vi "DAQ.Init.Override.vi"(8 "error in (no error)":errorcluster, 11 "DAQmx in":refnum<class "DAQmx.lvclass">) -> (0 "error out":errorcluster, 3 "DAQmx out":refnum<class "DAQmx.lvclass">)   [LabVIEW 2016, in "DAQmx.lvclass"]
uses:
  DAQmx.lvclass
  C:/user/patrick/hg/lockin.SMO/lvsrc/DAQ/DAQ.lvclass
  DAQ/DAQ.lvclass/DAQ.ctl
  DAQmx.lvclass/DAQmx.ctl
  <vilib>/DAQmx/write.llb/DAQmx Write (Analog 1D Wfm NChan NSamp).vi
  <vilib>/DAQmx/create/channels.llb/DAQmx Create Channel (AO-Voltage-Basic).vi
  <vilib>/DAQmx/create/channels.llb/DAQmx Create Channel (AI-Voltage-Basic).vi
  <vilib>/DAQmx/configure/timing.llb/DAQmx Timing (Sample Clock).vi
  <vilib>/DAQmx/miscellaneous.llb/DAQmx Fill In Error Info.vi
  <resource>/objmgr/daqmx.rc
  <vilib>/measure/NI_MABase.lvlib
  DAQ/DAQ.lvclass
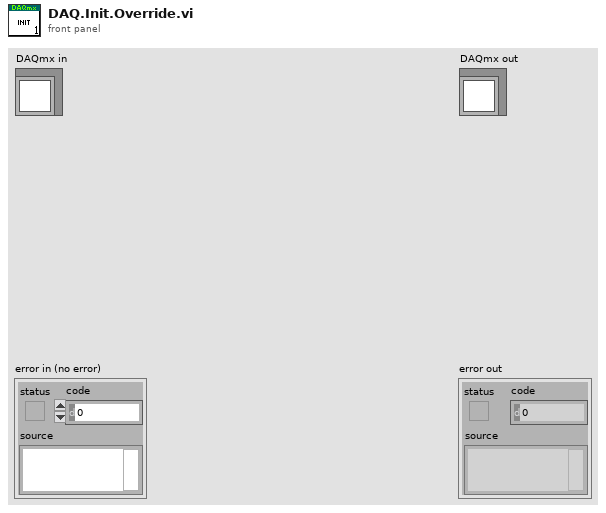
[diagram p1: front panel]
types:
  T1 = typedef "DAQ.lvclass/PrivateEvents--DAQ.AO.Channels.ctl" = string
  T2 = typedef "DAQ.lvclass/PrivateEvents--DAQ.AI.Channels.ctl" = string
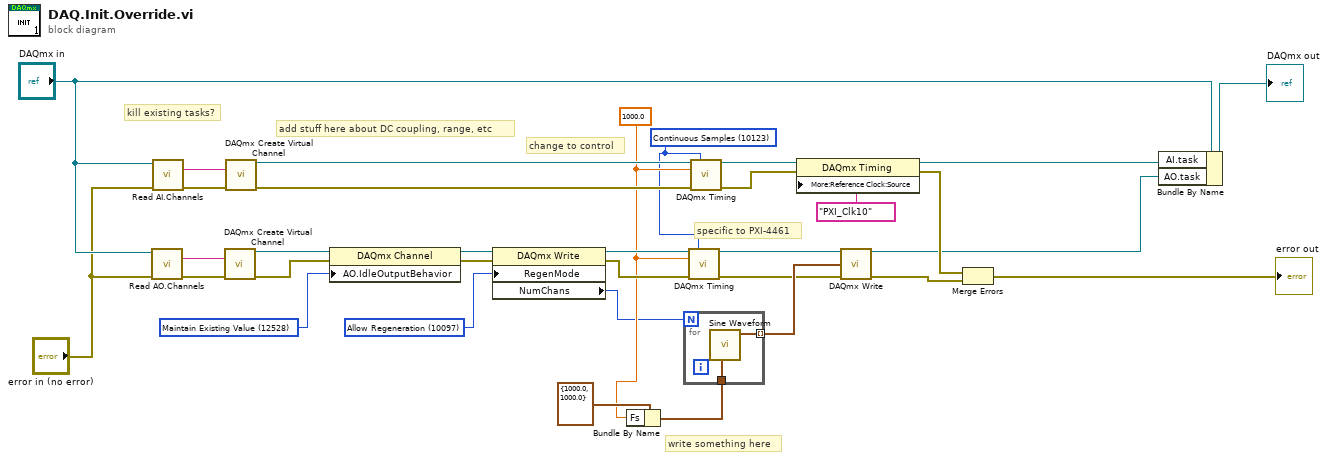
[diagram p0: block diagram]
diagram:
  w1 = 10123 items=["Finite Samples"=10178, "Continuous Samples"=10123, "Hardware Timed Single Point"=12522] ("sample mode")
  w3 = 10097 items=["Allow Regeneration"=10097, "Do Not Allow Regeneration"=10158] ("RegenMode")
  w4 = 12528 items=["Zero Volts"=12526, "High-Impedance"=12527, "Maintain Existing Value"=12528] ("AO.IdleOutputBehavior")
  w5 = 1000.0 ("rate")
  # "kill existing tasks?"
  # "write something here"
  # "add stuff here about DC coupling, range, etc"
  # "specific to PXI-4461"
  # "change to control"
  n1 = call "Read AO.Channels.vi"("error in (no error)"="error in (no error)", "DAQ in"="DAQmx in") -> ("error out"=w7:errorcluster, "AO.Channels"=w9:T1)  [unwired: 7 in, 1 out]
  n2 = call "Read AI.Channels.vi"("error in (no error)"="error in (no error)", "DAQ in"="DAQmx in") -> ("error out"=w6:errorcluster, "AI.Channels"=w10:T2)  [unwired: 7 in, 1 out]
  n3 = call-poly <vilib>:"DAQmx Create Virtual Channel.vi"("physical channels"=w9, "error in"=w7) -> ("task out"=w27:refnum<k21>, "error out"=w26:errorcluster)  [unwired: 12 in]
  n4 = call-poly <vilib>:"DAQmx Create Virtual Channel.vi"("physical channels"=w10, "error in"=w6) -> ("task out"=w32:refnum<k21>, "error out"=w31:errorcluster)  [unwired: 12 in]
  n5 = property class="DAQmx Channel"(reference=w27, error in=w26, "AO.IdleOutputBehavior"=w4) -> (reference out=w28:refnum<k21>, error out=w29:errorcluster)
  n6 = property class="DAQmx Write"(reference=w28, error in=w29, "RegenMode"=w3) -> (reference out=w25:refnum<k21>, error out=w24:errorcluster, "NumChans"=w2:u32)
  n7 = Bundle By Name(cluster=cluster{"Fs":dbl, "#s":dbl} {"Fs"=1000.0, "#s"=1000.0} ("sampling info"), "Fs"=w5) -> (w21:cluster{"Fs":dbl, "#s":dbl})
  n8 = for {
    N: w2 -> [_]
    tunnel: w21 -> [w35]
    tunnel: [w34] -> w20 mode=indexing
    n9 = call <vilib>:"Sine Waveform.vi"("sampling info"=w35) -> ("signal out"=w34:waveform(dbl))  [unwired: 9 in, 1 out]
  }
  n10 = call-poly <vilib>:"DAQmx Timing.vi"("task/channels in"=w25, "sample mode"=w1, "rate"=w5, "error in"=w24) -> ("task out"=w23:refnum<k21>, "error out"=w19:errorcluster)  [unwired: 10 in]
  n11 = call-poly <vilib>:"DAQmx Timing.vi"("task/channels in"=w32, "sample mode"=w1, "rate"=w5, "error in"=w31) -> ("task out"=w33:refnum<k21>, "error out"=w18:errorcluster)  [unwired: 10 in]
  n12 = property class="DAQmx Timing"(reference=w33, error in=w18, "More:Reference Clock:Source"=tag "PXI_Clk10" ("RefClk.Src")) -> (reference out=w13:refnum<k21>, error out=w17:errorcluster)
  n13 = call-poly <vilib>:"DAQmx Write.vi"("task/channels in"=w23, "data"=w20, "error in"=w19) -> ("task out"=w14:refnum<k21>, "error out"=w16:errorcluster)  [unwired: 10 in, 1 out]
  n14 = Merge Errors(w17, w16) -> (→"error out":errorcluster)
  n15 = Bundle By Name(cluster="DAQmx in", "AI.task"=w13, "AO.task"=w14) -> (→"DAQmx out":refnum<class "DAQmx.lvclass">)
